vi "Main.vi"() -> ()   [LabVIEW 2020]
doc: "Machine d'état première partie"
uses:
  Controller/Ctrl_Display.ctl
  Controller/Ctrl_enum_state.ctl
  Controller/Ctrl_Local.ctl
  Controller/Ctrl_operateur.ctl
panel:
  in  "Btn_Arrêter":bool
  out "Ind_Display":T1
  in  "Cmd_Operateur":T2
  in  "Cmd_Pad":T3
  out "error out":errorcluster caption="sortie d'erreur"
  in  "error in":errorcluster caption="entrée d'erreur"
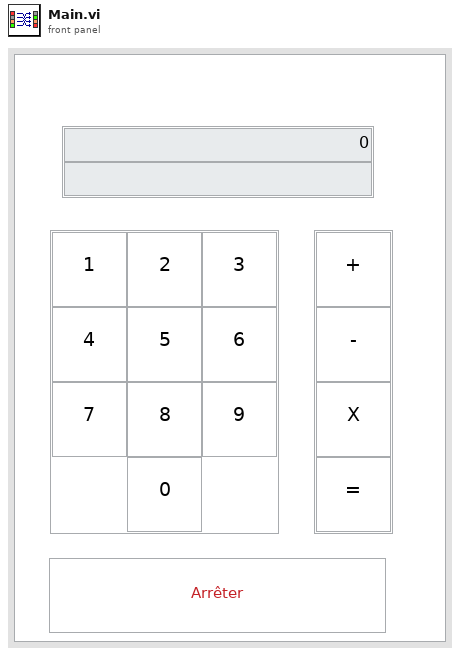
[diagram p1: front panel]
types:
  T1 = typedef "Ctrl_Display.ctl" = cluster{"Display_Numérique":dbl, "Display_Chaine":string}
  T2 = cluster{"Btn_+":bool, "Btn_-":bool, "Btn_X":bool, "Btn_=":bool}
  T3 = cluster{"Btn_1":bool, "Btn_2":bool, "Btn_3":bool, "Btn_4":bool, "Btn_5":bool, "Btn_6":bool, "Btn_7":bool, "Btn_8":bool, "Btn_9":bool, "Btn_10":bool}
  T4 = typedef "Ctrl_enum_state.ctl" = enum16{"Idle", "Init", "Display", "BTN_Num", "Exit"}
  T5 = typedef "Ctrl_Local.ctl" = cluster{"Operator":T6, "Ind_Display":T1, "Btn":i32, "State":T4}
  T6 = typedef "Ctrl_operateur.ctl" = enum16{"=", "*", "-", "+"}
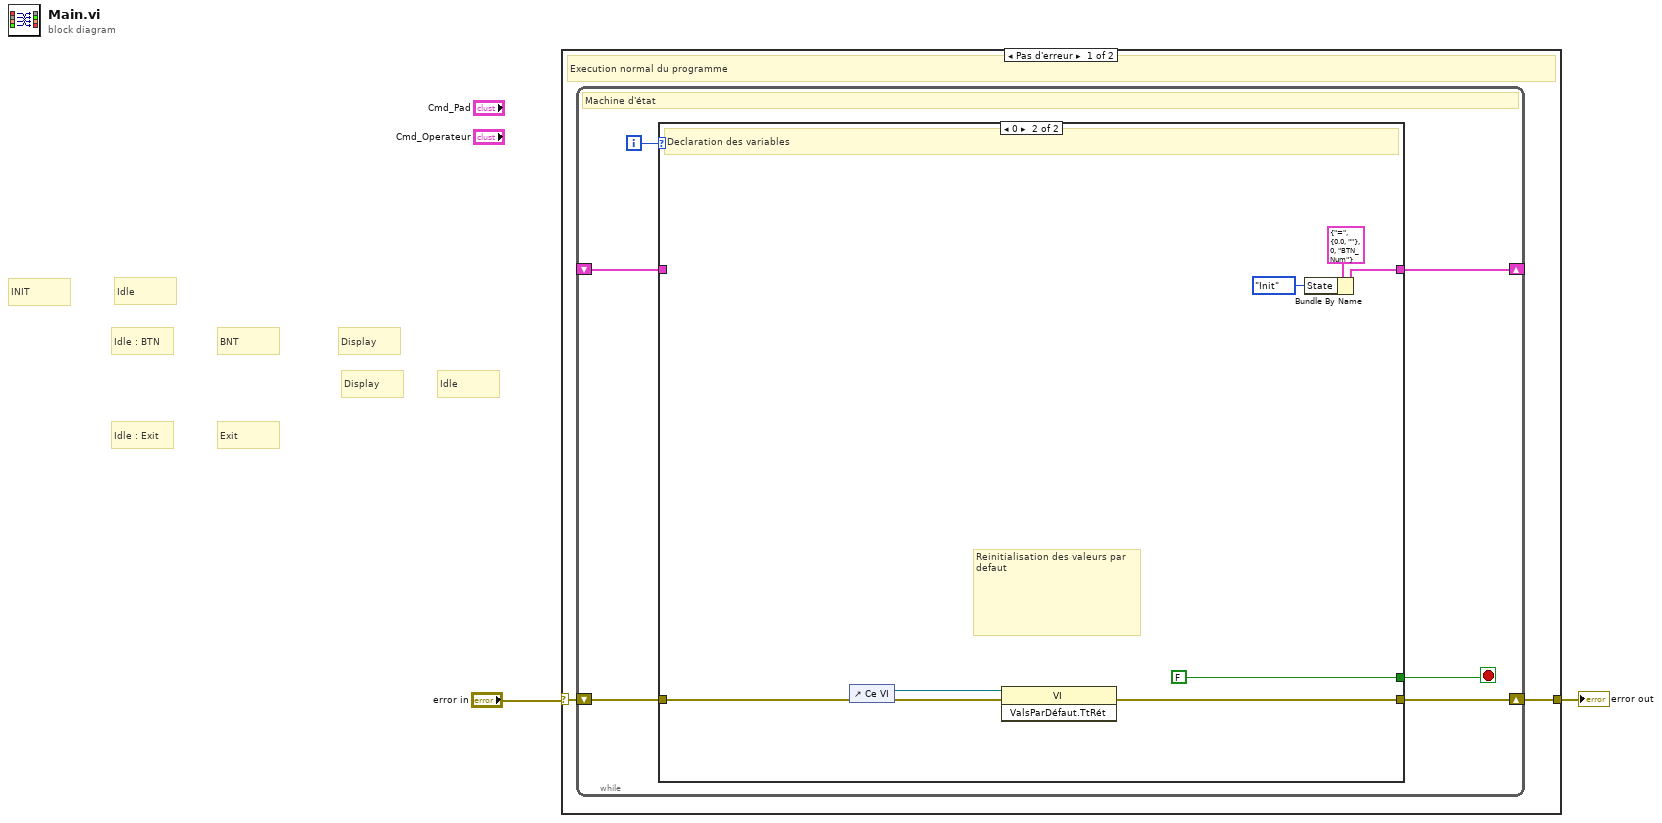
[diagram p0: block diagram]
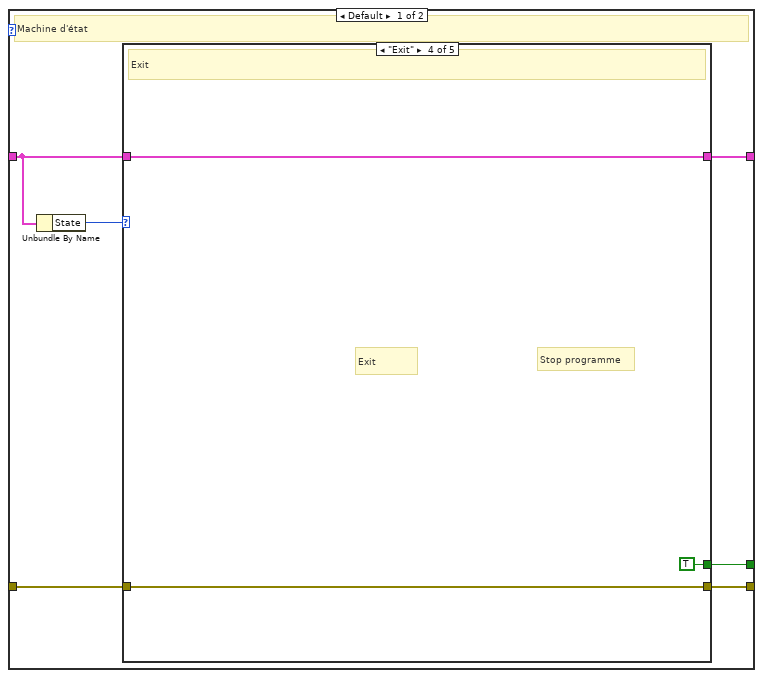
[diagram p2: hidden frame]
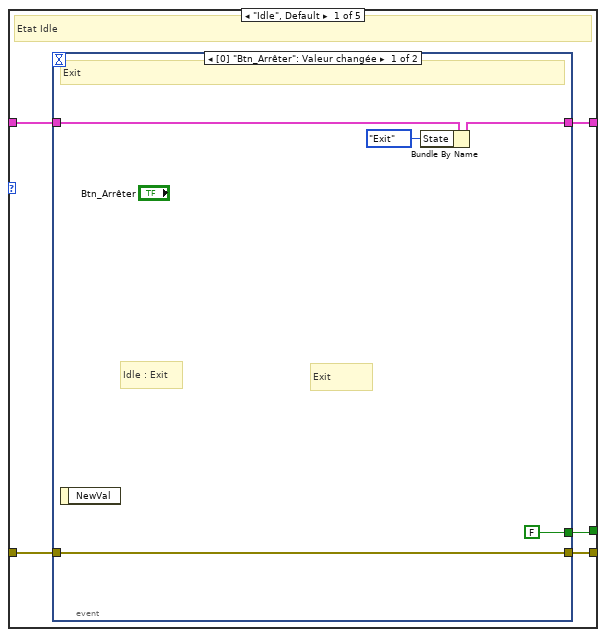
[diagram p3: hidden frame]
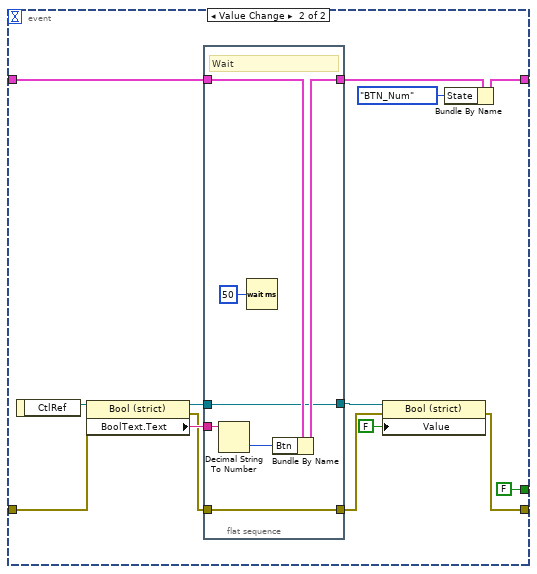
[diagram p4: hidden frame]
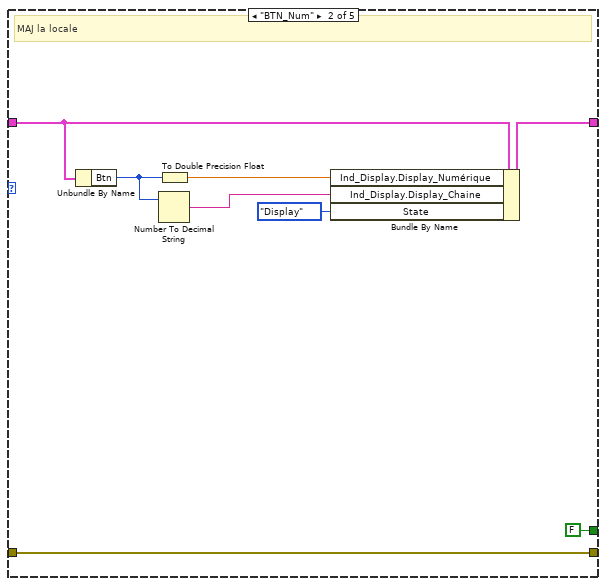
[diagram p5: hidden frame]
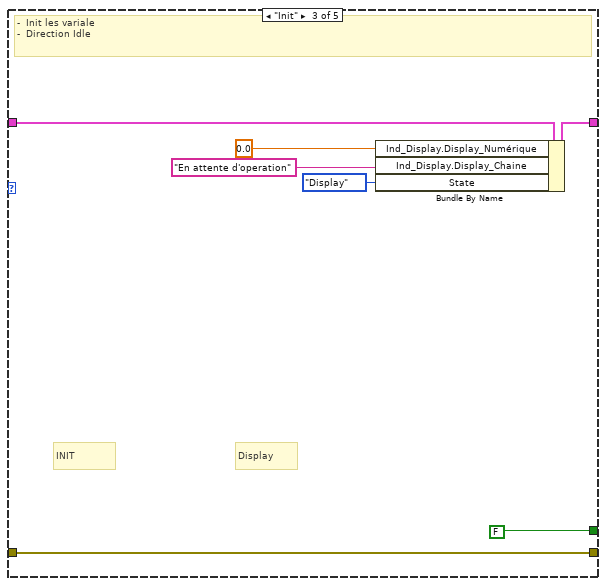
[diagram p6: hidden frame]
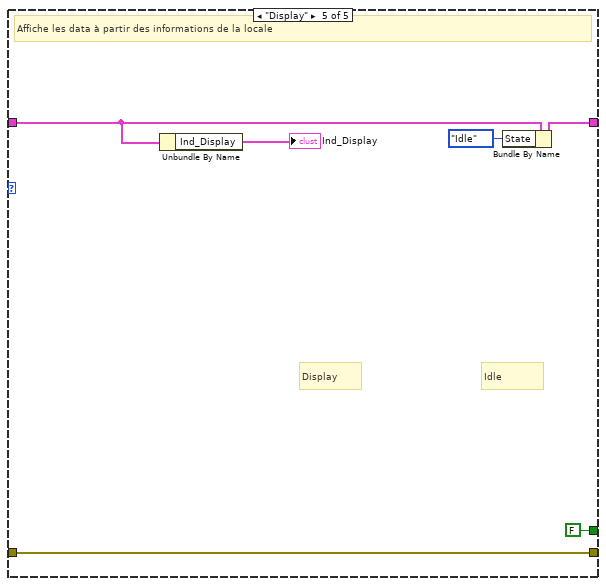
[diagram p7: hidden frame]
diagram:
  # "Display"
  # "Idle : BTN"
  # "BNT"
  # "Idle : Exit"
  # "Exit"
  # "Idle"
  # "INIT"
  # "Idle"
  # "Display"
  n1 = case shown="Pas d'erreur" "error in" {
    selector: "error in" -> [w4 w79]
    tunnel: [w3 w79] -> w1
    frame No Error {
      # "Execution normal du programme"
      n2 = while {
        shift-right: [w9] -> w3
        shift-left: w4 -> [w10]
        shift-right: [w6] -> _
        shift-left: _ -> [w5]
        i -> [w8]
        stop <- w7 stop-if-true
        # "Machine d'état"
        n3 = case shown="0" w8 {
          tunnel: w10 -> [w15 w75]
          tunnel: [w14 w74] -> w9
          tunnel: [w13 FALSE] -> w7
          tunnel: [w16 w73] -> w6
          tunnel: w5 -> [w12 _]
          frame Default {
            # "Machine d'état"
            n4 = Unbundle By Name(w12) -> ("State"=w11:T4)
            n5 = case shown="\"Exit\"" w11 {
              tunnel: w12 -> [w21 w52 w62 w63 w71]
              tunnel: [w20 w53 w61 w63 w67] -> w16
              tunnel: w15 -> [w19 w55 w60 w65 w70]
              tunnel: [w18 w55 w60 w65 w70] -> w14
              tunnel: [w17 FALSE FALSE TRUE FALSE] -> w13
              frame "Idle", Default {
                # "Etat Idle"
                n6 = event shown="[0] \"Btn_Arrêter\": Valeur changée" {
                  selector: _ -> [_ _]
                  dyn-events: _ -> [_ _]
                  timeout: _ -> [_ _]
                  tunnel: w21 -> [w24 w39]
                  tunnel: [w23 w28] -> w20
                  tunnel: w19 -> [w26 w36]
                  tunnel: [w26 w30] -> w18
                  tunnel: [FALSE FALSE] -> w17
                  event "Btn_Arrêter": Value Change {
                    # "Exit"
                    # "Idle : Exit"
                    # "Exit"
                    n7 = event-data() -> ()  [unwired: 1 in, 1 out]
                    n8 = Bundle By Name(cluster=w24, "State"=Ctrl_enum_state."Exit") -> (w23:T5)
                  }
                  event "Cmd_Pad.Btn_1", "Cmd_Pad.Btn_2", "Cmd_Pad.Btn_3", "Cmd_Pad.Btn_4", "Cmd_Pad.Btn_5", "Cmd_Pad.Btn_6", "Cmd_Pad.Btn_7", "Cmd_Pad.Btn_8", "Cmd_Pad.Btn_9", "Cmd_Pad.Btn_10": Value Change {
                    n9 = event-data() -> ("CtlRef"=w37:refnum<vi>)  [unwired: 1 in]
                    n10 = property class="Bool (strict)"(reference=w37, error in=w36) -> (reference out=w34:refnum<vi>, error out=w33:errorcluster, "BoolText.Text"=w35:string)
                    n11 = flat-sequence {
                      tunnel: w39 -> [w47]
                      tunnel: [w46] -> w38
                      tunnel: w35 -> [w45]
                      tunnel: w34 -> [w43]
                      tunnel: [w43] -> w32
                      tunnel: w33 -> [w42]
                      tunnel: [w42] -> w31
                      frame #0 {
                        # "Wait"
                        n12 = Decimal String To Number(string=w45) -> (number=w44:i32)  [unwired: 2 in, 1 out]
                        n13 = Wait (ms)(milliseconds to wait=u32 50 ("attente (ms)")) -> ()  [unwired: 1 out]
                        n14 = Bundle By Name(cluster=w47, "Btn"=w44) -> (w46:T5)
                      }
                    }
                    n15 = property class="Bool (strict)"(reference=w32, error in=w31, "Value"=FALSE ("Valeur")) -> (error out=w30:errorcluster)  [unwired: 1 out]
                    n16 = Bundle By Name(cluster=w38, "State"=Ctrl_enum_state."BTN_Num") -> (w28:T5)
                  }
                }
              }
              frame "BTN_Num" {
                # "MAJ la locale"
                n17 = Unbundle By Name(w52) -> ("Btn"=w50:i32)
                n18 = Number To Decimal String(number=w50) -> (decimal integer string=w49:string)  [unwired: 1 in]
                n19 = To Double Precision Float(number=w50) -> (double precision float=w51:dbl)
                n20 = Bundle By Name(cluster=w52, "Ind_Display.Display_Numérique"=w51, "Ind_Display.Display_Chaine"=w49, "State"=Ctrl_enum_state."Display") -> (w53:T5)
              }
              frame "Init" {
                # "Display"
                # "INIT"
                # "-  Init les variale \n-  Direction Idle"
                n21 = Bundle By Name(cluster=w62, "Ind_Display.Display_Numérique"=0.0 ("Display_Numérique"), "Ind_Display.Display_Chaine"="En attente d'operation" ("Display_Chaine"), "State"=Ctrl_enum_state."Display") -> (w61:T5)
              }
              frame "Exit" {
                # "Stop programme"
                # "Exit"
                # "Exit"
              }
              frame "Display" {
                # "Idle"
                # "Display"
                # "Affiche les data à partir des informations de la locale"
                n22 = Unbundle By Name(w71) -> ("Ind_Display"=→"Ind_Display":T1)
                n23 = Bundle By Name(cluster=w71, "State"=Ctrl_enum_state."Idle") -> (w67:T5)
              }
            }
          }
          frame 0 {
            # "Reinitialisation des valeurs par defaut"
            # "Declaration des variables"
            n24 = control-ref of="Ce VI"() -> (w76:refnum<vi>)
            n25 = invoke class="VI" method="ValsParDéfaut.TtRét"(reference=w76, error in=w75) -> (error out=w74:errorcluster)  [unwired: 1 in, 2 out]
            n26 = Bundle By Name(cluster=T5 {"Operator"=enum."=", "Ind_Display"={"Display_Numérique"=0.0, "Display_Chaine"=""}, "Btn"=0, "State"=enum."BTN_Num"} ("Declaration_Local"), "State"=Ctrl_enum_state."Init") -> (w73:T5)
          }
        }
      }
    }
    frame Error {
      # "Erreur on laisse passer le flux"
    }
  }
  "error out" <- w1
